vi "ImageQDummy.vi"(8 "error in (no error)":errorcluster, 11 "Image in":refnum<class "Image.lvclass">) -> (0 "error out":errorcluster, 3 "Image out":refnum<class "Image.lvclass">)   [LabVIEW 2012, in "Image.lvclass"]
uses:
  classes/Image.lvclass
  classes/Image.lvclass/Image.ctl
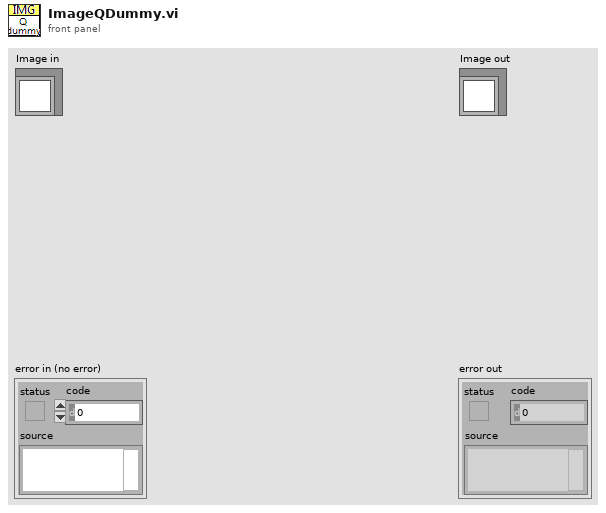
[diagram p1: front panel]
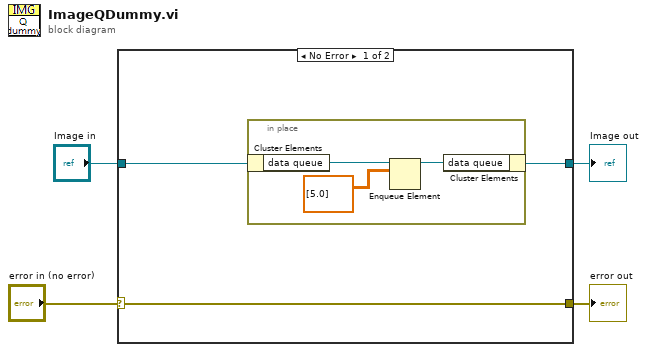
[diagram p0: block diagram]
diagram:
  n1 = case shown="No Error" "error in (no error)" {
    selector: "error in (no error)" -> [w7 w12]
    tunnel: [w7 w12] -> w3
    tunnel: [w6 w11] -> w1
    tunnel: "Image in" -> [w5 w11]
    frame No Error {
      n2 = in-place {
        n3 = in-place-cluster #1(w5) -> ("data queue"=w9:refnum<queue>)
        n4 = Enqueue Element(queue=w9, element=dbl[][] [[5.0]]) -> (queue out=w10:refnum<queue>)  [unwired: 2 in, 2 out]
        n5 = in-place-cluster #1("data queue"=w10) -> (w6:refnum<class "Image.lvclass">)
      }
    }
    frame Error {
    }
  }
  "error out" <- w3
  "Image out" <- w1
